vi "Fill Control.vi"(7 "PID gains":T2={"proportional gain (Kc)"=1.0, "integral time (Ti, min)"=0.0, "derivative time (Td, min)"=0.0} {"derivative time (Td, min)" format="%.3f"; "integral time (Ti, min)" format="%.3f"; "proportional gain (Kc)" format="%.3f"}, 8 "Fill Cutoff Pressure":dbl[unit], 9 "Manifold Pressure":dbl[unit], 10 "Fill State":T1(ring)=enum."Diluent Fill", 11 "Hold State":T1(ring)=enum."Diluent Fill") -> (2 "Valve Open?":bool, 3 "Output State":T1(ring))   [LabVIEW 2018]
uses:
  <vilib>/addons/control/pid/pid.llb/PID (DBL).vi
  <vilib>/addons/control/pid/NI_PID_pid.lvlib
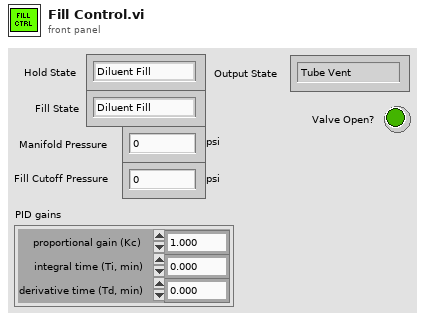
[diagram p1: front panel]
types:
  T1 = enum16{"Tube Vent", "Mix Section Purge", "Tube Purge", "Tube Vacuum", "Diluent Fill", "Oxidizer Fill", "Fuel Fill", "Fill Hold", "Mixing", "Tube Closed", "Ignition", "Manifold Vent"}
  T2 = cluster{"proportional gain (Kc)":dbl, "integral time (Ti, min)":dbl, "derivative time (Td, min)":dbl}
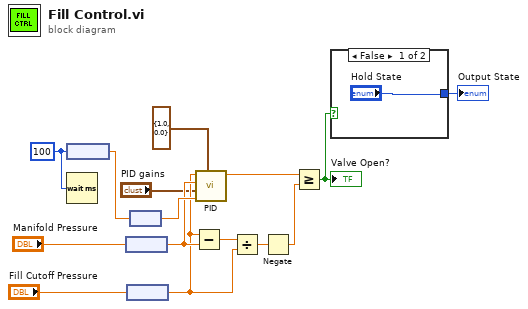
[diagram p0: block diagram]
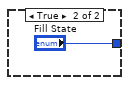
[diagram p2: hidden frame]
diagram:
  w13 = u32 100 ("milliseconds to wait")
  n1 = node(w13) -> (w15:dbl[unit])
  n2 = Wait (ms)(milliseconds to wait=w13) -> ()  [unwired: 1 out]
  n3 = node("Manifold Pressure") -> (w10:dbl)
  n4 = node("Fill Cutoff Pressure") -> (w5:dbl)
  n5 = node(w15) -> (w14:dbl)
  n6 = Subtract(x=w5, y=w10) -> (x-y=w7:dbl)
  n7 = call-poly <vilib>:"PID.vi"("output range"=cluster{"output high":dbl, "output low":dbl} {"output high"=1.0, "output low"=0.0}, "dt (s)"=w14, "PID gains"="PID gains", "process variable"=w10, "setpoint"=w5) -> ("output"=w9:dbl)  [unwired: 5 in, 1 out]
  n8 = Divide(x=w7, y=w5) -> (x/y=w6:dbl)
  n9 = Negate(x=w6) -> (-x=w8:dbl)
  n10 = Greater Or Equal?(x=w9, y=w8) -> (x >= y?=w11:bool)
  "Valve Open?" <- w11
  n11 = case shown="False" w11 {
    tunnel: ["Hold State" "Fill State"] -> w1
    frame False {
    }
    frame True {
    }
  }
  "Output State" <- w1
